vi "FRIC_navX_Get_LinearAcceleration.vi"(5 "Device Number":T1, 7 "Update":bool) -> (2 "Linear Acceleration":T2)   [LabVIEW 2016]
doc: "This navX VI returns the linear acceleration from the navX."
uses:
  _TypeDefs/FRIC_navX_DeviceNumbersTypeDef.ctl
  _TypeDefs/Z900_navX_DeviceRegisters.ctl
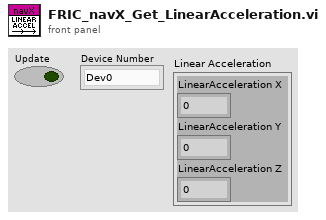
[diagram p1: front panel]
types:
  T1 = typedef "FRIC_navX_DeviceNumbersTypeDef.ctl" = enum16{"Dev0", "Dev1", "Dev2", "Dev3", "Dev4", "Dev5", "Dev6", "Dev7", "Dev8", "Dev9", "Dev10"}
  T2 = cluster{"LinearAcceleration X":dbl, "LinearAcceleration Y":dbl, "LinearAcceleration Z":dbl}
  T3 = typedef "Z900_navX_DeviceRegisters.ctl" = u8
  T4 = cluster{"LinearAcceleration X":dbl, "LinearAcceleration Y":dbl, "LinearAcceleration Z":dbl}[]
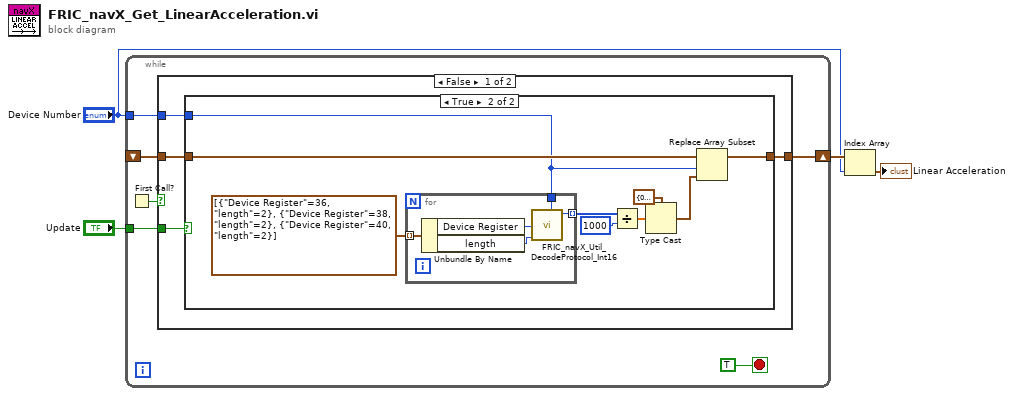
[diagram p0: block diagram]
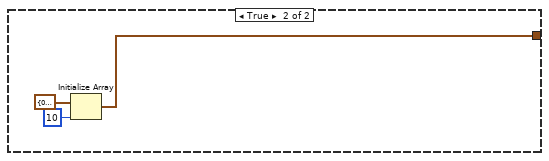
[diagram p3: hidden frame]
diagram:
  n1 = while {
    shift-right: [w10] -> w3
    shift-left: _ -> [w7]
    tunnel: "Update" -> [w8]
    tunnel: "Device Number" -> [w5]
    stop <- TRUE stop-if-true
    n2 = First Call?() -> (First Call?: T/F=w6:bool)
    n3 = case shown="False" w6 {
      tunnel: [w14 w30] -> w10
      tunnel: w8 -> [w11 _]
      tunnel: w7 -> [w13 _]
      tunnel: w5 -> [w12 _]
      frame False {
        n4 = case shown="True" w11 {
          tunnel: [w15 w18] -> w14
          tunnel: w13 -> [w15 w19]
          tunnel: w12 -> [_ w16]
          frame False {
          }
          frame True {
            n5 = for {
              tunnel: cluster{"Device Register":T3, "length":i32}[] [{"Device Register"=36, "length"=2}, {"Device Register"=38, "length"=2}, {"Device Register"=40, "length"=2}] ("Array") -> [w27] mode=indexing
              tunnel: [w26] -> w21 mode=indexing
              tunnel: w16 -> [w25]
              n6 = Unbundle By Name(w27) -> ("Device Register"=w29:T3, "length"=w28:i32)
              n7 = call "FRIC_navX_Util_DecodeProtocol_Int16.vi"("Device Number"=w25, "length"=w28, "Device Register"=w29) -> ("Value"=w26:i16)  [unwired: 8 in]
            }
            n8 = Divide(x=w21, y=1000) -> (x/y=w20:dbl[])
            n9 = Type Cast(type=T2 {"LinearAcceleration X"=0.0, "LinearAcceleration Y"=0.0, "LinearAcceleration Z"=0.0}, x=w20) -> (*(type *) &x=w17:T2)
            n10 = Replace Array Subset(array=w19, new element=w17, index=w16) -> (w18:T4)
          }
        }
      }
      frame True {
        n11 = Initialize Array(T2 {"LinearAcceleration X"=0.0, "LinearAcceleration Y"=0.0, "LinearAcceleration Z"=0.0}, 10 ("dimension size")) -> (w30:T4)
      }
    }
  }
  n12 = Index Array(array=w3, index="Device Number") -> (element=→"Linear Acceleration":T2)
